vi "Update signal cluster array.vi"(9 "Data in":dbl[](array[numeric]), 10 "Angle M2":dbl, 11 "Signals":cluster{"Signal":cluster{"X":dbl, "Y":dbl}[]}[](array[cluster])) -> (1 "Data out":dbl, 2 "Cluster":cluster{"X":dbl, "Y":dbl}, 3 "Array":cluster{"Array":cluster{"X":dbl, "Y":dbl}[]}[](array[cluster]))   [LabVIEW 2020]
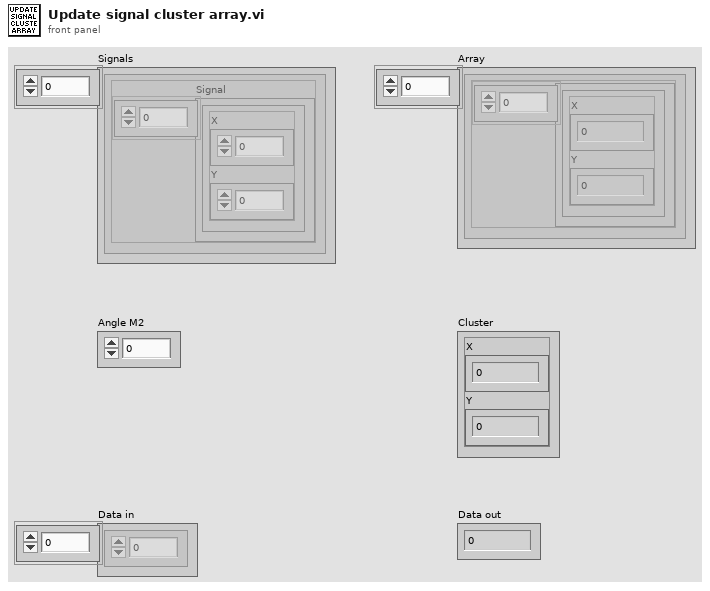
[diagram p1: front panel]
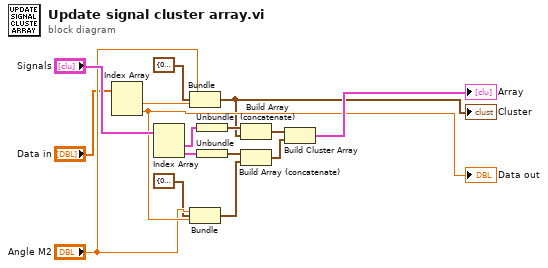
[diagram p0: block diagram]
diagram:
  n1 = Index Array(array="Data in") -> (element #1=w4:dbl, element #2=w7:dbl)  [unwired: 2 in]
  "Data out" <- w7
  n2 = Index Array(array="Signals") -> (element #1=w9:cluster{"Signal":cluster{"X":dbl, "Y":dbl}[]}, element #2=w16:cluster{"Signal":cluster{"X":dbl, "Y":dbl}[]})  [unwired: 2 in]
  n3 = Bundle(cluster=cluster{"X":dbl, "Y":dbl} {"X"=0.0, "Y"=0.0}, "X"="Angle M2", "Y"=w4) -> (w3:cluster{"X":dbl, "Y":dbl})
  "Cluster" <- w3
  n4 = Bundle(cluster=cluster{"X":dbl, "Y":dbl} {"X"=0.0, "Y"=0.0}, "X"="Angle M2", "Y"=w7) -> (w12:cluster{"X":dbl, "Y":dbl})
  n5 = Unbundle(w9) -> ("Signal"=w10:cluster{"X":dbl, "Y":dbl}[])
  n6 = Unbundle(w16) -> ("Signal"=w11:cluster{"X":dbl, "Y":dbl}[])
  n7 = Build Array (concatenate)(w10, w3) -> (w13:cluster{"X":dbl, "Y":dbl}[])
  n8 = Build Array (concatenate)(w11, w12) -> (w14:cluster{"X":dbl, "Y":dbl}[])
  n9 = Build Cluster Array(w13, w14) -> (→"Array":cluster{cluster{"X":dbl, "Y":dbl}[]}[])
